vi "1A Interpret NMEA Sentence.vi"(11 "NMEA Sentence":string) -> ()   [LabVIEW 2013]
doc: "Interprets the NMEA 0813 sentences that we are using from our Airmar PB200 WeatherStation sensor.\nBy Jaime McCandless\nTODO: finish implementing NMEA sentences"
uses:
  <vilib>/regexp/Match Regular Expression.xnode
  2-Think/2 Globals/2 Global.vi
  2-Think/2 Typedefs/Velocity.ctl
  2-Think/2 Typedefs/apparent wind.ctl
  2-Think/2 Typedefs/pitch and roll.ctl
  2-Think/2 Typedefs/heading.ctl
  Data/TypeDefs/UTM Location.ctl
panel:
  in  "UTC Time Zone":i32=-5
  in  "Tab Control":T1(tab)
  out "GPS (GGA) Data":T2
  out "GPS (GLL) Data":T3
  out "GPGSA Data":T4
  out "UTC Time":timestamp
  out "Local Time":timestamp
  out "Lattitude (ddmm.mmmm)":dbl format="%_8g"
  out "Lattitude North/South":string
  out "Longitude (ddmm.mmmm)":dbl format="%_8g"
  out "Longitude East/West":string
  out "Speed over ground (knots)":dbl format="%_3g"
  out "Course over ground (degrees)":dbl format="%_4g"
  out "Magnetic Variation (degrees)":dbl format="%_4g"
  out "Variation East/West":string
  out "GPS (RMC) Data":T5 {"Course over ground (degrees)" format="%#.6g"; "Speed over ground (knots)" format="%#.6g"; "Magnetic Variation (degrees)" format="%#.6g"; "Longitude (ddmm.mmmm)" format="%#.6g"; "Lattitude (ddmm.mmmm)" format="%#.6g"}
  out "GPS Data Valid?":bool
  out "Robot UTM Location":T6 {"North" format="%#_10f"; "East" format="%#_8f"}
  out "GPS (VTG) Data":T7
  out "Heading":dbl
  out "Turn (ROT) Data":T8
  out "Meteorological Data":T9
  out "Theoretical true wind direction":T10(graph)
  out "Relative wind direction":cluster{dbl, "Filtered Value Out":dbl}(graph)
  out "Wind (MWV) Data, Theoretical":T11
  out "Wind (MWV) Data, Relative":T11
  out "Transducer (XDR) B Data":cluster{"Pitch (deg)":dbl, "Roll (deg)":dbl}
  out "Transducer (XDR) A Data":T12
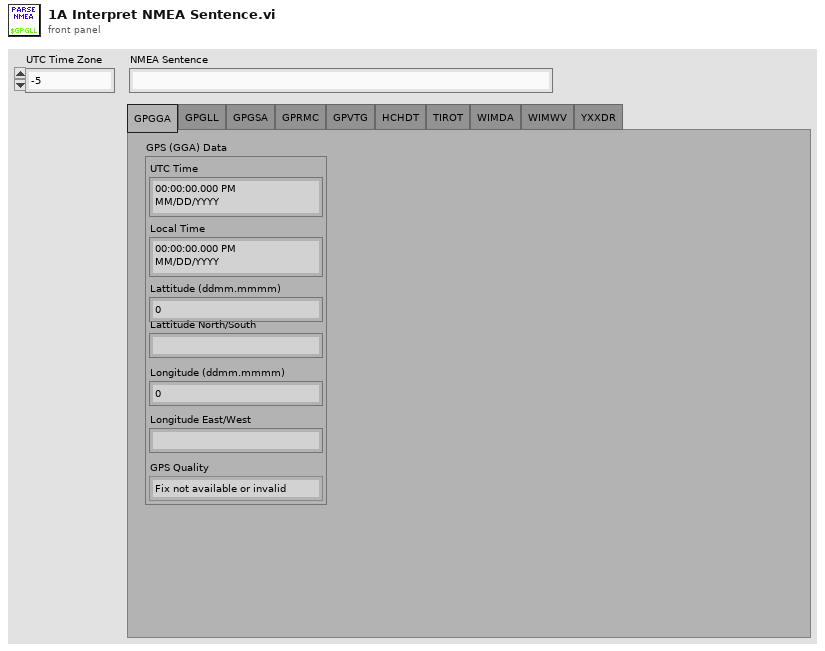
[diagram p1: front panel]
types:
  T1 = enum32{"GPGGA", "GPGLL", "GPGSA", "GPRMC", "GPVTG", "HCHDT", "TIROT", "WIMDA", "WIMWV", "YXXDR"}
  T2 = cluster{"UTC Time":timestamp, "Local Time":timestamp, "Lattitude (ddmm.mmmm)":dbl, "Lattitude North/South":string, "Longitude (ddmm.mmmm)":dbl, "Longitude East/West":string, "GPS Quality":enum16{"Fix not available or invalid", "GPS SPS Mode, fix valid", "Differential GPS, SPS Mode, fix valid", "GPS PPS Mode, fix valid", "Real Time Kinematic (RTK)", "Float RTK", "Estimated (dead reckoning) Mode", "Manual Input Mode", "Simulator Mode"}}
  T3 = cluster{"UTC Time":timestamp, "Local Time":timestamp, "Lattitude (ddmm.mmmm)":dbl, "Lattitude North/South":string, "Longitude (ddmm.mmmm)":dbl, "Longitude East/West":string, "GPS Mode":string, "GPS Data Valid?":bool}
  T4 = cluster{"Mode":string, "Fix Strength":i32, "Satellite IDs":i32[], "PDOP":dbl, "HDOP":dbl, "VDOP":dbl}
  T5 = cluster{"UTC Time":timestamp, "Local Time":timestamp, "Lattitude (ddmm.mmmm)":dbl, "Lattitude North/South":string, "Longitude (ddmm.mmmm)":dbl, "Longitude East/West":string, "Magnetic Variation (degrees)":dbl, "Variation East/West":string, "Speed over ground (knots)":dbl, "Course over ground (degrees)":dbl}
  T6 = typedef "UTM Location.ctl" = cluster{"UTM Zone":dbl, "Hemisphere":enum16{"North", "South"}, "East":dbl, "North":dbl}
  T7 = cluster{"Course Over Ground (True)":dbl, "Course Over Ground (Magnetic)":dbl, "Speed Over Ground (Knots)":dbl, "Speed Over Ground (km/hr)":dbl, "GPS Mode":string}
  T8 = cluster{"Rate of Turn (deg/min)":dbl, "Turn Rotation Data Valid?":bool}
  T9 = cluster{"Barometric Pressure (inches of mercury)":dbl, "Barometric Pressure (bars)":dbl, "Air temperature (degC)":dbl, "Relative humidity (%)":dbl, "Wind direction, True (deg)":dbl, "Wind direction, Magnetic (deg)":dbl, "Wind speed (knots)":dbl, "Wind speed (m/s)":dbl}
  T10 = cluster{"Robot\nHeading ":dbl, "Robot\nHeading ":dbl}
  T11 = cluster{"Angle relative to boat (deg)":dbl, "Wind Data Valid?":bool, "Wind speed (knots)":dbl, "True (T) or Relative (R)":string}
  T12 = cluster{"Calc. Relative Wind Chill (degC)":dbl, "Calc. Theoretical Wind Chill (degC)":dbl, "Calc. Heat Index (degC)":dbl, "Meas. Barometric Pressure (bars)":dbl}
  T13 = cluster{"second":i32, "minute":i32, "hour":i32, "day of month":i32, "month":i32, "year":i32, "day of week":i32, "day of year":i32, "is DST":i32}
  T14 = typedef "heading.ctl" = dbl
  T15 = typedef "Velocity.ctl" = cluster{"East":dbl, "North":dbl}
  T16 = typedef "apparent wind.ctl" = cluster{"Toward Fore":dbl, "Toward Starboard":dbl}
  T17 = typedef "pitch and roll.ctl" = cluster{"Pitch":dbl, "Roll":dbl}
  T18 = typedef "generalized sensor status.ctl" = cluster{"Sensor Connected":T19, "Sensor Initialized":T19, "Sensor OK":T19, "Latest Error String":string, "GPS Lock":T19}
  T19 = typedef "indicator LED.ctl" = bool
  T20 = cluster{"BoatVelocityInY":dbl, "BoatVelocityInX":dbl}
  T21 = cluster{"Robot\nHeading ":T14, "Robot\nHeading ":T14}
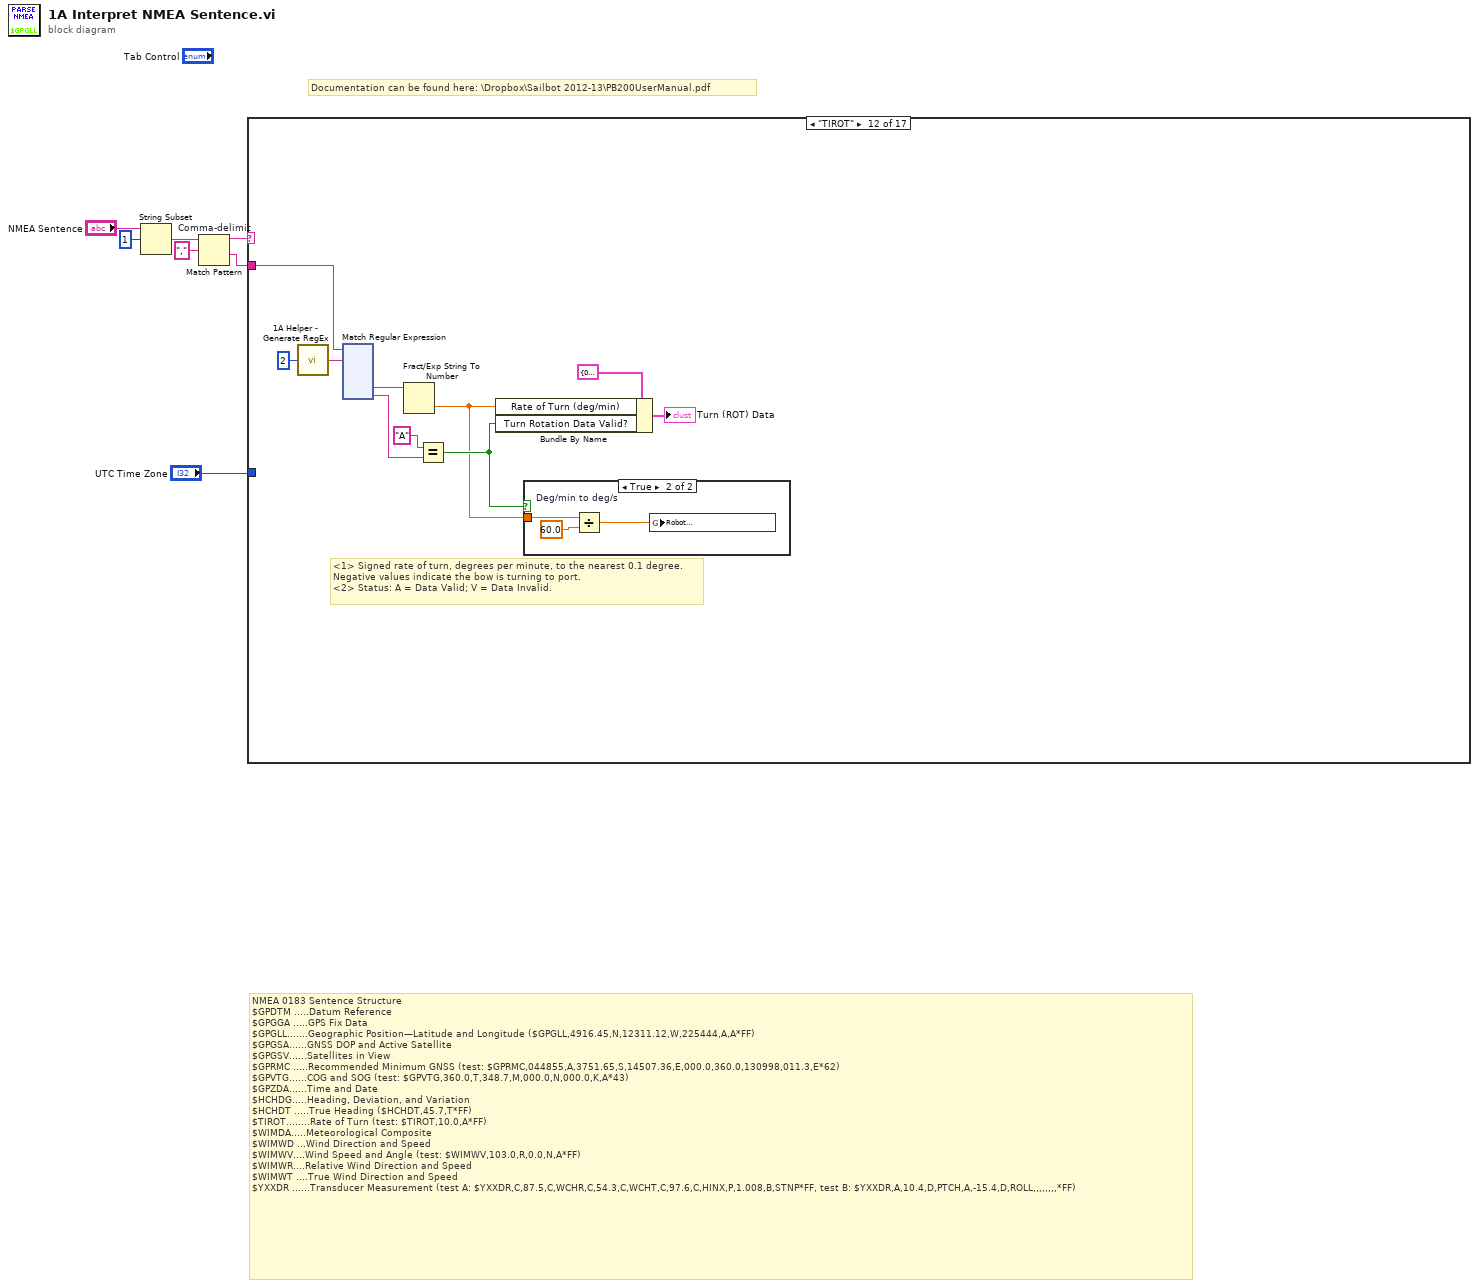
[diagram p0: block diagram]
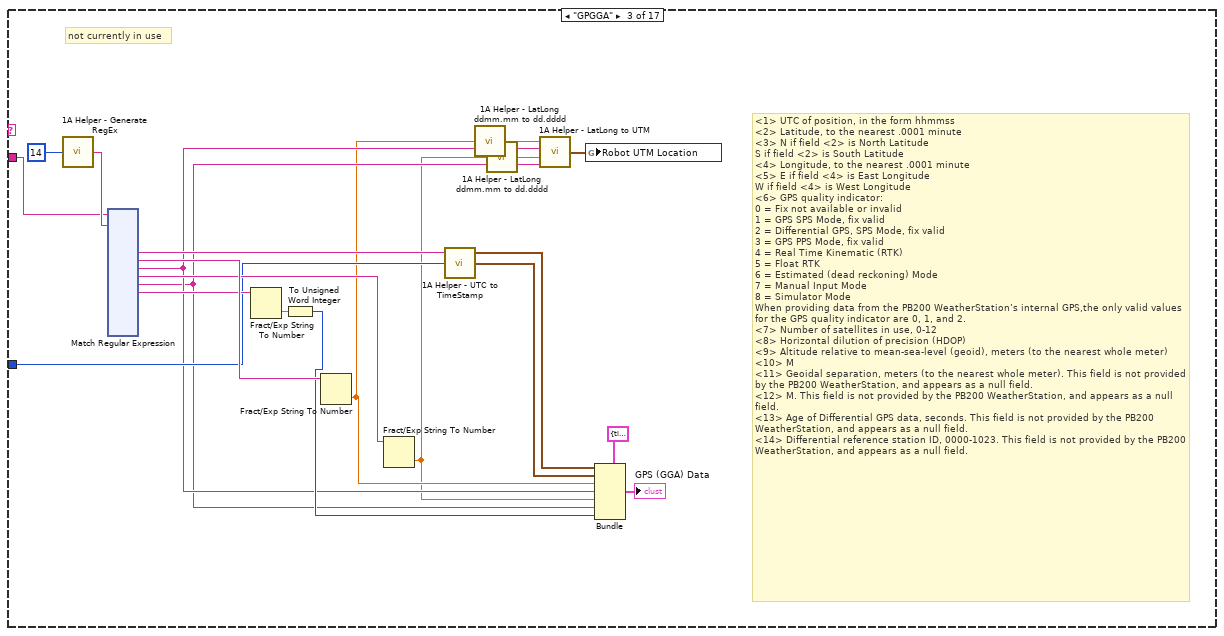
[diagram p4: hidden frame]
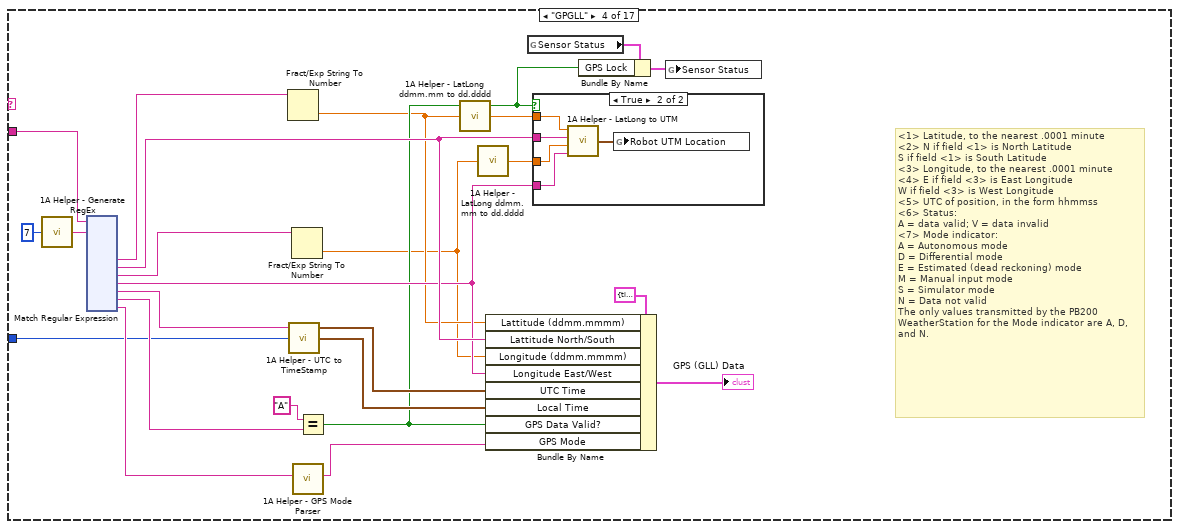
[diagram p5: hidden frame]
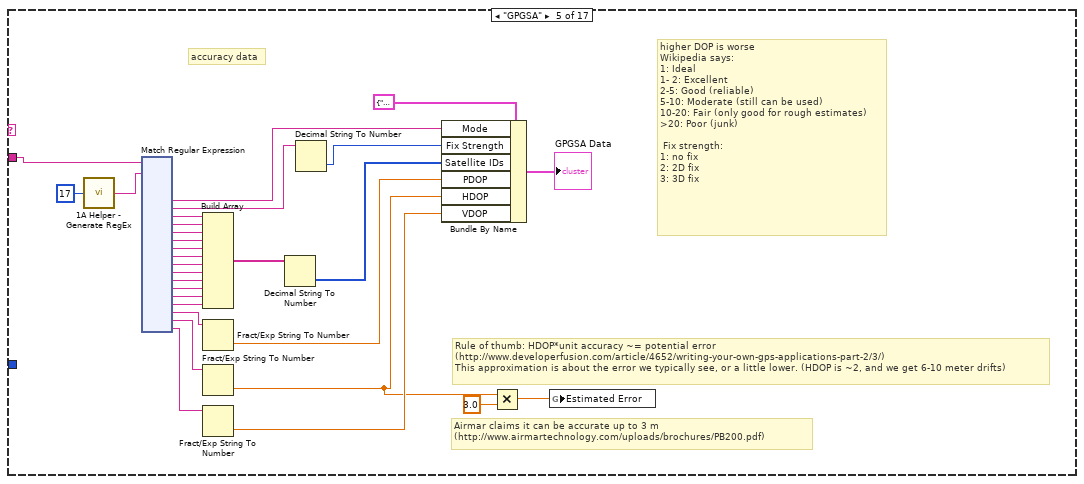
[diagram p7: hidden frame]
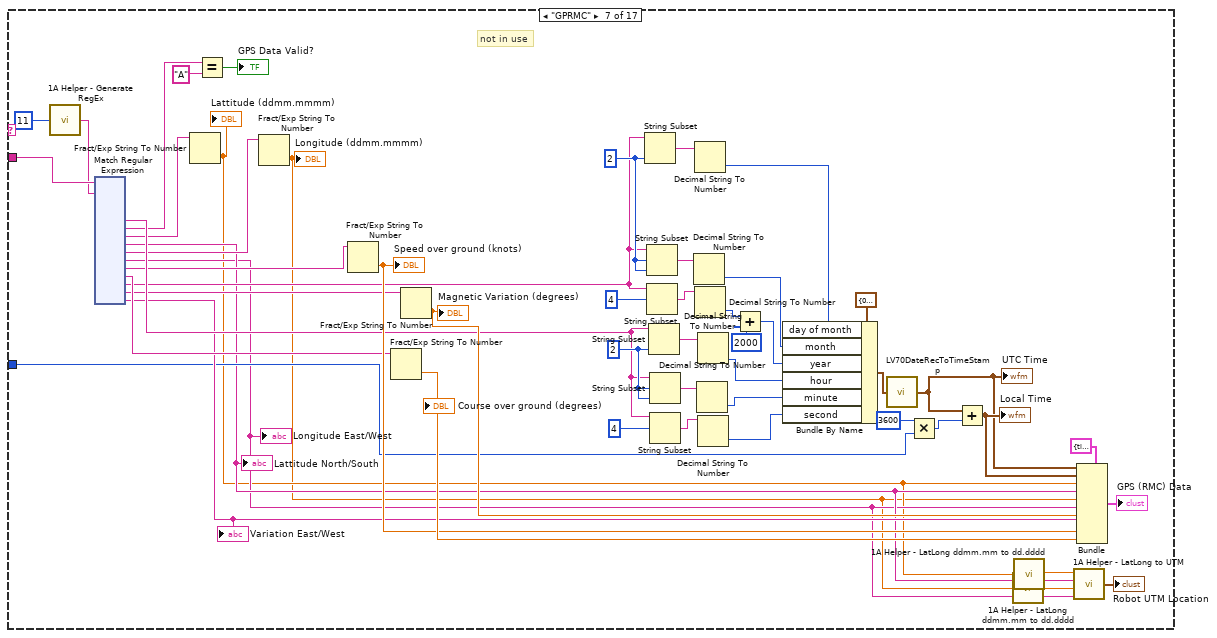
[diagram p9: hidden frame]
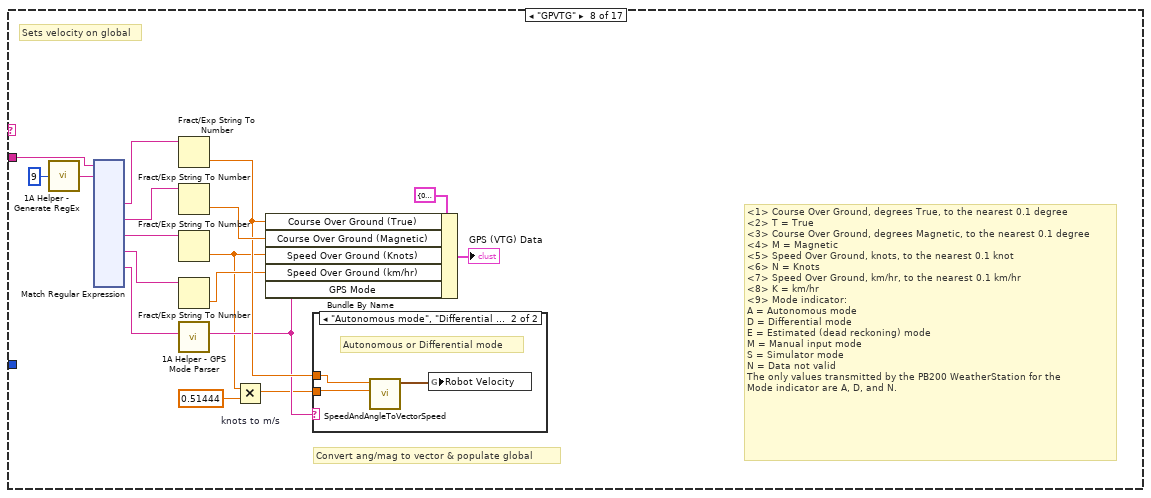
[diagram p10: hidden frame]
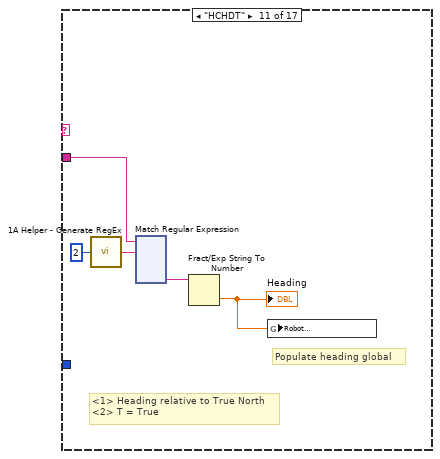
[diagram p14: hidden frame]
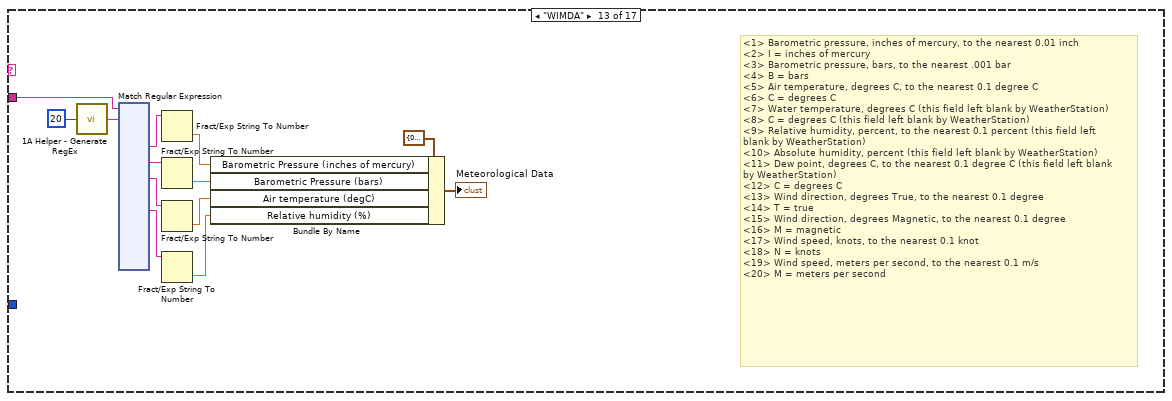
[diagram p16: hidden frame]
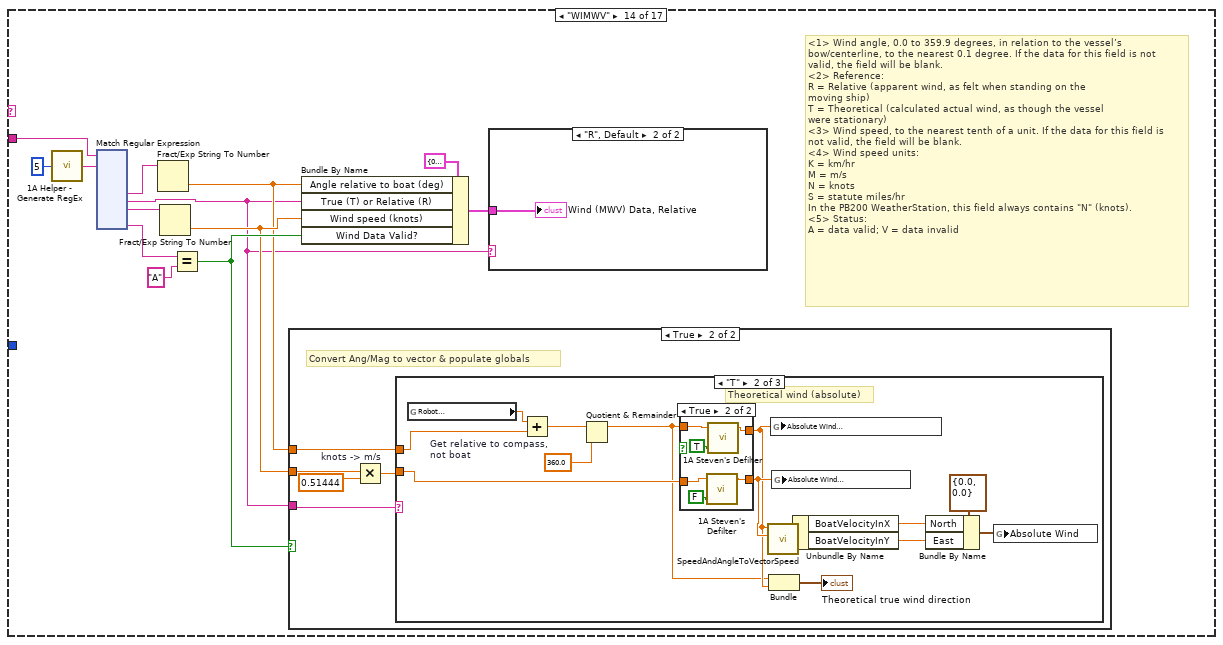
[diagram p17: hidden frame]
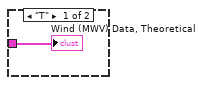
[diagram p18: hidden frame]
diagram:
  # "Documentation can be found here: \\Dropbox\\Sailbot 2012-13\\PB200UserManual.pdf"
  # "NMEA 0183 Sentence Structure\n$GPDTM .....Datum Reference\n$GPGGA .....GPS Fix Data\n$GPGLL.......Geographic Position—Latitude and Longitude ($GPGLL,4916.45,N,12311.12,W,225444,A,A*FF)\n$GPGSA......GNSS DOP and Active Satellite\n$GPGSV......Satellites in View\n$GPRMC .....Recommended Minimum GNSS (test: $GPRMC,044855,A,3751.65,S,14507.36,E,000.0,360.0,130998,011.3,E*62)\n$GPVTG......COG and SOG (test: $GPVTG,360.0,T,348.7,M,000.0,N,000.0,K,A*43)\n$GPZDA......Time and Date\n$HCHDG.....Heading, Deviation, and Variation\n$HCHDT .....True Heading ($HCHDT,45.7,T*FF)\n$TIROT........Rate of Turn (test: $TIROT,10.0,A*FF)\n$WIMDA.....Meteorological Composite\n$WIMWD ...Wind Direction and Speed\n$WIMWV....Wind Speed and Angle (test: $WIMWV,103.0,R,0.0,N,A*FF)\n$WIMWR....Relative Wind Direction and Speed\n$WIMWT ....True Wind Direction and Speed\n$YXXDR ......Transducer Measurement (test A: $YXXDR,C,87.5,C,WCHR,C,54.3,C,WCHT,C,97.6,C,HINX,P,1.008,B,STNP*FF, test B: $YXXDR,A,10.4,D,PTCH,A,-15.4,D,ROLL,,,,,,,,*FF)"
  n1 = String Subset(string="NMEA Sentence", offset (0)=1) -> (substring=w4:string)  [unwired: 1 in]
  n2 = Match Pattern "Comma-delimit"(string=w4, regular expression=",") -> (before substring=w5:string, after substring=w6:string)  [unwired: 1 in, 2 out]
  n3 = case shown="\"TIROT\"" w5 {
    tunnel: w6 -> [_ _ w26 w170 w329 _ w478 w647 _ _ w778 w900 w1031 w1170 _ _ w1329]
    tunnel: "UTC Time Zone" -> [_ _ w15 w162 _ _ w466 _ _ _ _ _ _ _ _ _ _]
    frame "", Default {
    }
    frame "GPDTM" {
      # "unimplemented"
    }
    frame "GPGGA" {
      # "not currently in use"
      # "<1> UTC of position, in the form hhmmss\n<2> Latitude, to the nearest .0001 minute\n<3> N if field <2> is North Latitude\nS if field <2> is South Latitude\n<4> Longitude, to the nearest .0001 minute\n<5> E if field <4> is East Longitude\nW if field <4> is West Longitude\n<6> GPS quality indicator:\n0 = Fix not available or invalid\n1 = GPS SPS Mode, fix valid\n2 = Differential GPS, SPS Mode, fix valid\n3 = GPS PPS Mode, fix valid\n4 = Real Time Kinematic (RTK)\n5 = Float RTK\n6 = Estimated (dead reckoning) Mode\n7 = Manual Input Mode\n8 = Simulator Mode\nWhen providing data from the PB200 WeatherStation’s internal GPS,the only valid values for the GPS quality indicator are 0, 1, and 2.\n<7> Number of satellites in use, 0-12\n<8> Horizontal dilution of precision (HDOP)\n<9> Altitude relative to mean-sea-level (geoid), meters (to the nearest whole meter)\n<10> M\n<11> Geoidal separation, meters (to the nearest whole meter). This field is not provided by the PB200 WeatherStation, and appears as a null field.\n<12> M. This field is not provided by the PB200 WeatherStation, and appears as a null field.\n<13> Age of Differential GPS data, seconds. This field is not provided by the PB200 WeatherStation, and appears as a null field.\n<14> Differential reference station ID, 0000-1023. This field is not provided by the PB200 WeatherStation, and appears as a null field."
      n4 = call "1A Helper - Generate RegEx.vi"("# Datums"=14) -> ("RegEx"=w27:string)
      n5 = xnode "Match Regular Expression"("input string"=w26, "regular expression"=w27) -> ("submatch 1"=w18:string, "submatch 2"=w24:string, "submatch 3"=w13:string, "submatch 4"=w23:string, "submatch 5"=w12:string, "submatch 6"=w22:string)  [unwired: 4 in, 10 out]
      n6 = Fract/Exp String To Number(string=w22) -> (number=w21:dbl)  [unwired: 3 in, 1 out]
      n7 = To Unsigned Word Integer(number=w21) -> (unsigned 16bit integer=w20:u16)
      n8 = Fract/Exp String To Number(string=w24) -> (number=w10:dbl)  [unwired: 3 in, 1 out]
      n9 = Fract/Exp String To Number(string=w23) -> (number=w8:dbl)  [unwired: 3 in, 1 out]
      n10 = call "1A Helper - UTC to TimeStamp.vi"("UTC Time Zone in"=w15, "UTC (hhmmss)"=w18) -> ("Local Time"=w16:timestamp, "UTC Time"=w17:timestamp)  [unwired: 2 in]
      n11 = call "1A Helper - LatLong ddmm.mm to dd.dddd.vi"("Lattitude/Longitude in ddmm.mmmm"=w10) -> ("Latitude/Longitude in dd.dddddd"=w11:dbl)
      n12 = call "1A Helper - LatLong ddmm.mm to dd.dddd.vi"("Lattitude/Longitude in ddmm.mmmm"=w8) -> ("Latitude/Longitude in dd.dddddd"=w9:dbl)
      n13 = call "1A Helper - LatLong to UTM.vi"("East/West"=w12, "Longitude"=w9, "North/South"=w13, "Latitude"=w11) -> ("Robot UTM Location"=w14:T6)
      n14 = global write "2 Global.vi" "Robot UTM Location"(w14) -> ()
      n15 = Bundle(cluster=T2 {"UTC Time"=timestamp(0 s since 1904-01-01), "Local Time"=timestamp(0 s since 1904-01-01), "Lattitude (ddmm.mmmm)"=0.0, "Lattitude North/South"="", "Longitude (ddmm.mmmm)"=0.0, "Longitude East/West"="", "GPS Quality"=enum."GPS SPS Mode, fix valid"} ("Cluster"), "UTC Time"=w17, "Local Time"=w16, "Lattitude (ddmm.mmmm)"=w10, "Lattitude North/South"=w13, "Longitude (ddmm.mmmm)"=w8, "Longitude East/West"=w12, "GPS Quality"=w20) -> (→"GPS (GGA) Data":T2)
    }
    frame "GPGLL" {
      # "<1> Latitude, to the nearest .0001 minute\n<2> N if field <1> is North Latitude\nS if field <1> is South Latitude\n<3> Longitude, to the nearest .0001 minute\n<4> E if field <3> is East Longitude\nW if field <3> is West Longitude\n<5> UTC of position, in the form hhmmss\n<6> Status:\nA = data valid; V = data invalid\n<7> Mode indicator:\nA = Autonomous mode\nD = Differential mode\nE = Estimated (dead reckoning) mode\nM = Manual input mode\nS = Simulator mode\nN = Data not valid\nThe only values transmitted by the PB200 WeatherStation for the Mode indicator are A, D, and N."
      n16 = call "1A Helper - Generate RegEx.vi"("# Datums"=7) -> ("RegEx"=w174:string)
      n17 = xnode "Match Regular Expression"("input string"=w170, "regular expression"=w174) -> ("submatch 1"=w173:string, "submatch 2"=w160:string, "submatch 3"=w172:string, "submatch 4"=w159:string, "submatch 5"=w169:string, "submatch 6"=w165:string, "submatch 7"=w171:string)  [unwired: 4 in, 5 out]
      n18 = Fract/Exp String To Number(string=w173) -> (number=w155:dbl)  [unwired: 3 in, 1 out]
      n19 = call "1A Helper - UTC to TimeStamp.vi"("UTC Time Zone in"=w162, "UTC (hhmmss)"=w169) -> ("Local Time"=w164:timestamp, "UTC Time"=w163:timestamp)  [unwired: 2 in]
      n20 = Fract/Exp String To Number(string=w172) -> (number=w153:dbl)  [unwired: 3 in, 1 out]
      n21 = call "1A Helper - GPS Mode Parser.vi"("GPS Mode (Char)"=w171) -> ("GPS Mode (Description)"=w167:string)  [unwired: 6 in]
      n22 = Equal?(x="A" ("y"), y=w165) -> (x = y?=w156:bool)
      n23 = call "1A Helper - LatLong ddmm.mm to dd.dddd.vi"("Lattitude/Longitude in ddmm.mmmm"=w155) -> ("Latitude/Longitude in dd.dddddd"=w154:dbl)
      n24 = call "1A Helper - LatLong ddmm.mm to dd.dddd.vi"("Lattitude/Longitude in ddmm.mmmm"=w153) -> ("Latitude/Longitude in dd.dddddd"=w152:dbl)
      n25 = Bundle By Name(cluster=T3 {"UTC Time"=timestamp(0 s since 1904-01-01), "Local Time"=timestamp(0 s since 1904-01-01), "Lattitude (ddmm.mmmm)"=0.0, "Lattitude North/South"="", "Longitude (ddmm.mmmm)"=0.0, "Longitude East/West"="", "GPS Mode"="", "GPS Data Valid?"=FALSE} ("Cluster"), "Lattitude (ddmm.mmmm)"=w155, "Lattitude North/South"=w160, "Longitude (ddmm.mmmm)"=w153, "Longitude East/West"=w159, "UTC Time"=w163, "Local Time"=w164, "GPS Data Valid?"=w156, "GPS Mode"=w167) -> (→"GPS (GLL) Data":T3)
      n26 = global read "2 Global.vi" "Sensor Status"() -> (w157:T18)
      n27 = case shown="True" w156 {
        tunnel: w154 -> [_ w180]
        tunnel: w160 -> [_ w179]
        tunnel: w152 -> [_ w178]
        tunnel: w159 -> [_ w177]
        frame False {
        }
        frame True {
          n28 = call "1A Helper - LatLong to UTM.vi"("East/West"=w177, "Longitude"=w178, "North/South"=w179, "Latitude"=w180) -> ("Robot UTM Location"=w176:T6)
          n29 = global write "2 Global.vi" "Robot UTM Location"(w176) -> ()
        }
      }
      n30 = Bundle By Name(cluster=w157, "GPS Lock"=w156) -> (w158:T18)
      n31 = global write "2 Global.vi" "Sensor Status"(w158) -> ()
    }
    frame "GPGSA" {
      # "Airmar claims it can be accurate up to 3 m\n(http://www.airmartechnology.com/uploads/brochures/PB200.pdf)"
      # "Rule of thumb: HDOP*unit accuracy ~= potential error\n(http://www.developerfusion.com/article/4652/writing-your-own-gps-applications-part-2/3/)\nThis approximation is about the error we typically see, or a little lower. (HDOP is ~2, and we get 6-10 meter drifts)"
      # "higher DOP is worse\nWikipedia says:\n1: Ideal\n1- 2: Excellent\n2-5: Good (reliable)\n5-10: Moderate (still can be used)\n10-20: Fair (only good for rough estimates)\n>20: Poor (junk)\n\n Fix strength: \n1: no fix\n2: 2D fix\n3: 3D fix"
      # "accuracy data"
      n32 = call "1A Helper - Generate RegEx.vi"("# Datums"=17) -> ("RegEx"=w328:string)
      n33 = xnode "Match Regular Expression"("input string"=w329, "regular expression"=w328) -> ("submatch 1"=w325:string, "submatch 2"=w324:string, "submatch 3"=w322:string, "submatch 4"=w321:string, "submatch 5"=w320:string, "submatch 6"=w319:string, "submatch 7"=w318:string, "submatch 8"=w317:string, "submatch 9"=w316:string, "submatch 10"=w315:string, "submatch 11"=w314:string, "submatch 12"=w313:string, "submatch 13"=w312:string, "submatch 14"=w311:string, "submatch 15"=w308:string, "submatch 16"=w306:string, "submatch 17"=w305:string)  [unwired: 4 in, 5 out]
      n34 = Build Array(w322, w321, w320, w319, w318, w317, w316, w315, w314, w313, w312, w311) -> (w310:string[])
      n35 = Fract/Exp String To Number(string=w308) -> (number=w307:dbl)  [unwired: 3 in, 1 out]
      n36 = Fract/Exp String To Number(string=w306) -> (number=w302:dbl)  [unwired: 3 in, 1 out]
      n37 = Fract/Exp String To Number(string=w305) -> (number=w304:dbl)  [unwired: 3 in, 1 out]
      n38 = Decimal String To Number(string=w310) -> (number=w309:i32[])  [unwired: 2 in, 1 out]
      n39 = Decimal String To Number(string=w324) -> (number=w323:i32)  [unwired: 2 in, 1 out]
      n40 = Bundle By Name(cluster=T4 {"Mode"="", "Fix Strength"=0, "Satellite IDs"=[], "PDOP"=0.0, "HDOP"=0.0, "VDOP"=0.0} ("GPGSA Data"), "Mode"=w325, "Fix Strength"=w323, "Satellite IDs"=w309, "PDOP"=w307, "HDOP"=w302, "VDOP"=w304) -> (→"GPGSA Data":T4)
      n41 = Multiply(x=w302, y=3.0) -> (x*y=w300:dbl)
      n42 = global write "2 Global.vi" "Estimated Error"(w300) -> ()
    }
    frame "GPGSV" {
      # "unimplemented"
    }
    frame "GPRMC" {
      w496 = 2 ("length (rest)")
      w486 = 2 ("length (rest)")
      # "not in use"
      n43 = call "1A Helper - Generate RegEx.vi"("# Datums"=11) -> ("RegEx"=w468:string)
      n44 = xnode "Match Regular Expression"("input string"=w478, "regular expression"=w468) -> ("submatch 1"=w477:string, "submatch 2"=w476:string, "submatch 3"=w475:string, "submatch 4"=w465:string, "submatch 5"=w474:string, "submatch 6"=w464:string, "submatch 7"=w473:string, "submatch 8"=w472:string, "submatch 9"=w471:string, "submatch 10"=w470:string, "submatch 11"=w469:string)  [unwired: 4 in, 5 out]
      "Lattitude North/South" <- w465
      "Longitude East/West" <- w464
      "Variation East/West" <- w469
      n45 = Fract/Exp String To Number(string=w475) -> (number=w461:dbl)  [unwired: 3 in, 1 out]
      "Lattitude (ddmm.mmmm)" <- w461
      n46 = Equal?(x=w476, y="A") -> (x = y?=→"GPS Data Valid?":bool)
      n47 = Fract/Exp String To Number(string=w474) -> (number=w459:dbl)  [unwired: 3 in, 1 out]
      "Longitude (ddmm.mmmm)" <- w459
      n48 = Fract/Exp String To Number(string=w473) -> (number=w506:dbl)  [unwired: 3 in, 1 out]
      "Speed over ground (knots)" <- w506
      n49 = Fract/Exp String To Number(string=w472) -> (number=w507:dbl)  [unwired: 3 in, 1 out]
      "Course over ground (degrees)" <- w507
      n50 = Fract/Exp String To Number(string=w470) -> (number=w505:dbl)  [unwired: 3 in, 1 out]
      "Magnetic Variation (degrees)" <- w505
      n51 = String Subset(string=w471, length (rest)=w496) -> (substring=w497:string)  [unwired: 1 in]
      n52 = String Subset(string=w471, offset (0)=w496, length (rest)=w496) -> (substring=w495:string)
      n53 = String Subset(string=w471, offset (0)=4) -> (substring=w493:string)  [unwired: 1 in]
      n54 = String Subset(string=w477, length (rest)=w486) -> (substring=w482:string)  [unwired: 1 in]
      n55 = String Subset(string=w477, offset (0)=w486, length (rest)=w486) -> (substring=w488:string)
      n56 = String Subset(string=w477, offset (0)=4) -> (substring=w490:string)  [unwired: 1 in]
      n57 = Decimal String To Number(string=w495) -> (number=w499:i32)  [unwired: 2 in, 1 out]
      n58 = Decimal String To Number(string=w497) -> (number=w498:i32)  [unwired: 2 in, 1 out]
      n59 = Decimal String To Number(string=w493) -> (number=w500:i32)  [unwired: 2 in, 1 out]
      n60 = Decimal String To Number(string=w488) -> (number=w487:i32)  [unwired: 2 in, 1 out]
      n61 = Decimal String To Number(string=w482) -> (number=w485:i32)  [unwired: 2 in, 1 out]
      n62 = Decimal String To Number(string=w490) -> (number=w491:i32)  [unwired: 2 in, 1 out]
      n63 = Add(x=w500, y=2000) -> (x+y=w502:i32)
      n64 = Bundle By Name(cluster=T13 {"second"=0, "minute"=0, "hour"=0, "day of month"=0, "month"=0, "year"=0, "day of week"=0, "day of year"=0, "is DST"=0} ("date time rec"), "day of month"=w498, "month"=w499, "year"=w502, "hour"=w485, "minute"=w487, "second"=w491) -> (w483:T13)
      n65 = call <vilib>:"LV70DateRecToTimeStamp.vi"("date time rec"=w483) -> ("Time Stamp"=w503:timestamp)
      "UTC Time" <- w503
      n66 = Multiply(x=3600 ("number"), y=w466) -> (x*y=w467:i32)
      n67 = Add(x=w503, y=w467) -> (x+y=w504:timestamp)
      "Local Time" <- w504
      n68 = call "1A Helper - LatLong ddmm.mm to dd.dddd.vi"("Lattitude/Longitude in ddmm.mmmm"=w459) -> ("Latitude/Longitude in dd.dddddd"=w460:dbl)
      n69 = call "1A Helper - LatLong ddmm.mm to dd.dddd.vi"("Lattitude/Longitude in ddmm.mmmm"=w461) -> ("Latitude/Longitude in dd.dddddd"=w462:dbl)
      n70 = call "1A Helper - LatLong to UTM.vi"("East/West"=w464, "Longitude"=w460, "North/South"=w465, "Latitude"=w462) -> ("Robot UTM Location"=→"Robot UTM Location":T6)
      n71 = Bundle(cluster=T5 {"UTC Time"=timestamp(0 s since 1904-01-01), "Local Time"=timestamp(0 s since 1904-01-01), "Lattitude (ddmm.mmmm)"=0.0, "Lattitude North/South"="", "Longitude (ddmm.mmmm)"=0.0, "Longitude East/West"="", "Magnetic Variation (degrees)"=0.0, "Variation East/West"="", "Speed over ground (knots)"=0.0, "Course over ground (degrees)"=0.0} ("Cluster"), "UTC Time"=w503, "Local Time"=w504, "Lattitude (ddmm.mmmm)"=w461, "Lattitude North/South"=w465, "Longitude (ddmm.mmmm)"=w459, "Longitude East/West"=w464, "Magnetic Variation (degrees)"=w505, "Variation East/West"=w469, "Speed over ground (knots)"=w506, "Course over ground (degrees)"=w507) -> (→"GPS (RMC) Data":T5)
    }
    frame "GPVTG" {
      # "Convert ang/mag to vector & populate global"
      # "Sets velocity on global"
      # "<1> Course Over Ground, degrees True, to the nearest 0.1 degree\n<2> T = True\n<3> Course Over Ground, degrees Magnetic, to the nearest 0.1 degree\n<4> M = Magnetic\n<5> Speed Over Ground, knots, to the nearest 0.1 knot\n<6> N = Knots\n<7> Speed Over Ground, km/hr, to the nearest 0.1 km/hr\n<8> K = km/hr\n<9> Mode indicator:\nA = Autonomous mode\nD = Differential mode\nE = Estimated (dead reckoning) mode\nM = Manual input mode\nS = Simulator mode\nN = Data not valid\nThe only values transmitted by the PB200 WeatherStation for the\nMode indicator are A, D, and N."
      n72 = call "1A Helper - Generate RegEx.vi"("# Datums"=9) -> ("RegEx"=w648:string)
      n73 = xnode "Match Regular Expression"("input string"=w647, "regular expression"=w648) -> ("submatch 1"=w644:string, "submatch 3"=w643:string, "submatch 5"=w641:string, "submatch 7"=w640:string, "submatch 9"=w639:string)  [unwired: 4 in, 11 out]
      n74 = Fract/Exp String To Number(string=w644) -> (number=w638:dbl)  [unwired: 3 in, 1 out]
      n75 = Fract/Exp String To Number(string=w643) -> (number=w642:dbl)  [unwired: 3 in, 1 out]
      n76 = Fract/Exp String To Number(string=w641) -> (number=w635:dbl)  [unwired: 3 in, 1 out]
      n77 = Fract/Exp String To Number(string=w640) -> (number=w637:dbl)  [unwired: 3 in, 1 out]
      n78 = call "1A Helper - GPS Mode Parser.vi"("GPS Mode (Char)"=w639) -> ("GPS Mode (Description)"=w636:string)  [unwired: 6 in]
      n79 = Multiply "knots to m/s"(x=w635, y=0.51444) -> (x*y=w634:dbl)
      n80 = Bundle By Name(cluster=T7 {"Course Over Ground (True)"=0.0, "Course Over Ground (Magnetic)"=0.0, "Speed Over Ground (Knots)"=0.0, "Speed Over Ground (km/hr)"=0.0, "GPS Mode"=""} ("GPS (VTG) Data 2"), "Course Over Ground (True)"=w638, "Course Over Ground (Magnetic)"=w642, "Speed Over Ground (Knots)"=w635, "Speed Over Ground (km/hr)"=w637, "GPS Mode"=w636) -> (→"GPS (VTG) Data":T7)
      n81 = case shown="\"Autonomous mode\", \"Differential mode\"" w636 {
        tunnel: w638 -> [_ w652]
        tunnel: w634 -> [_ w651]
        frame "Data not valid", Default {
          # "Data not valid"
        }
        frame "Autonomous mode", "Differential mode" {
          # "Autonomous or Differential mode"
          n82 = call "SpeedAndAngleToVectorSpeed.vi"("BoatSpeed (m/s)"=w651, "RobotHeading (deg)"=w652) -> ("BoatVectorVelocity"=w650:T20)  [unwired: 9 in]
          n83 = global write "2 Global.vi" "Robot Velocity"(w650) -> ()
        }
      }
    }
    frame "GPZDA" {
      # "<1> UTC time of day, in the form hhmmss\n<2> UTC day, 01 to 31\n<3> UTC month, 01 to 12\n<4> UTC year (four digits, e.g. 2006)\n<5> Local time zone hours, 00 to +/-13 hrs\n<6> Local time zone minutes, 00 to +59"
    }
    frame "HCHDG " {
      # "<1> Magnetic sensor heading, degrees, to the nearest 0.1 degree.\n<2> Magnetic deviation, degrees east or west, to the nearest 0.1 degree.\n<3> E if field <2> is degrees East\nW if field <2> is degrees West\n<4> Magnetic variation, degrees east or west, to the nearest 0.1 degree.\n<5> E if field <4> is degrees East\nW if field <4> is degrees West"
    }
    frame "HCHDT" {
      # "Populate heading global"
      # "<1> Heading relative to True North\n<2> T = True"
      n84 = call "1A Helper - Generate RegEx.vi"("# Datums"=2) -> ("RegEx"=w779:string)
      n85 = xnode "Match Regular Expression"("input string"=w778, "regular expression"=w779) -> ("submatch 1"=w777:string)  [unwired: 4 in, 5 out]
      n86 = Fract/Exp String To Number(string=w777) -> (number=w776:dbl)  [unwired: 3 in, 1 out]
      "Heading" <- w776
      n87 = global write "2 Global.vi" "Robot\nHeading"(w776) -> ()
    }
    frame "TIROT" {
      # "<1> Signed rate of turn, degrees per minute, to the nearest 0.1 degree.\nNegative values indicate the bow is turning to port.\n<2> Status: A = Data Valid; V = Data Invalid."
      n88 = call "1A Helper - Generate RegEx.vi"("# Datums"=2) -> ("RegEx"=w902:string)
      n89 = xnode "Match Regular Expression"("input string"=w900, "regular expression"=w902) -> ("submatch 1"=w901:string, "submatch 2"=w896:string)  [unwired: 4 in, 5 out]
      n90 = Fract/Exp String To Number(string=w901) -> (number=w894:dbl)  [unwired: 3 in, 1 out]
      n91 = Equal?(x="A" ("y"), y=w896) -> (x = y?=w895:bool)
      n92 = Bundle By Name(cluster=T8 {"Rate of Turn (deg/min)"=0.0, "Turn Rotation Data Valid?"=TRUE} ("Turn (ROT) Data 2"), "Rate of Turn (deg/min)"=w894, "Turn Rotation Data Valid?"=w895) -> (→"Turn (ROT) Data":T8)
      n93 = case shown="True" w895 {
        tunnel: w894 -> [_ w905]
        frame False {
        }
        frame True {
          n94 = Divide "Deg/min to deg/s"(x=w905, y=60.0) -> (x/y=w906:dbl)
          n95 = global write "2 Global.vi" "Robot\nRate of Turn"(w906) -> ()
        }
      }
    }
    frame "WIMDA" {
      # "<1> Barometric pressure, inches of mercury, to the nearest 0.01 inch\n<2> I = inches of mercury\n<3> Barometric pressure, bars, to the nearest .001 bar\n<4> B = bars\n<5> Air temperature, degrees C, to the nearest 0.1 degree C\n<6> C = degrees C\n<7> Water temperature, degrees C (this field left blank by WeatherStation)\n<8> C = degrees C (this field left blank by WeatherStation)\n<9> Relative humidity, percent, to the nearest 0.1 percent (this field left\nblank by WeatherStation)\n<10> Absolute humidity, percent (this field left blank by WeatherStation)\n<11> Dew point, degrees C, to the nearest 0.1 degree C (this field left blank\nby WeatherStation)\n<12> C = degrees C\n<13> Wind direction, degrees True, to the nearest 0.1 degree\n<14> T = true\n<15> Wind direction, degrees Magnetic, to the nearest 0.1 degree\n<16> M = magnetic\n<17> Wind speed, knots, to the nearest 0.1 knot\n<18> N = knots\n<19> Wind speed, meters per second, to the nearest 0.1 m/s\n<20> M = meters per second"
      n96 = call "1A Helper - Generate RegEx.vi"("# Datums"=20) -> ("RegEx"=w1032:string)
      n97 = xnode "Match Regular Expression"("input string"=w1031, "regular expression"=w1032) -> ("submatch 1"=w1025:string, "submatch 3"=w1024:string, "submatch 5"=w1023:string, "submatch 9"=w1022:string)  [unwired: 4 in, 17 out]
      n98 = Fract/Exp String To Number(string=w1025) -> (number=w1029:dbl)  [unwired: 3 in, 1 out]
      n99 = Fract/Exp String To Number(string=w1024) -> (number=w1028:dbl)  [unwired: 3 in, 1 out]
      n100 = Fract/Exp String To Number(string=w1023) -> (number=w1027:dbl)  [unwired: 3 in, 1 out]
      n101 = Fract/Exp String To Number(string=w1022) -> (number=w1026:dbl)  [unwired: 3 in, 1 out]
      n102 = Bundle By Name(cluster=T9 {"Barometric Pressure (inches of mercury)"=0.0, "Barometric Pressure (bars)"=0.0, "Air temperature (degC)"=0.0, "Relative humidity (%)"=0.0, "Wind direction, True (deg)"=0.0, "Wind direction, Magnetic (deg)"=0.0, "Wind speed (knots)"=0.0, "Wind speed (m/s)"=0.0} ("Meteorological Data"), "Barometric Pressure (inches of mercury)"=w1029, "Barometric Pressure (bars)"=w1028, "Air temperature (degC)"=w1027, "Relative humidity (%)"=w1026) -> (→"Meteorological Data":T9)
    }
    frame "WIMWV" {
      # "<1> Wind angle, 0.0 to 359.9 degrees, in relation to the vessel’s\nbow/centerline, to the nearest 0.1 degree. If the data for this field is not\nvalid, the field will be blank.\n<2> Reference:\nR = Relative (apparent wind, as felt when standing on the\nmoving ship)\nT = Theoretical (calculated actual wind, as though the vessel\nwere stationary)\n<3> Wind speed, to the nearest tenth of a unit. If the data for this field is\nnot valid, the field will be blank.\n<4> Wind speed units:\nK = km/hr\nM = m/s\nN = knots\nS = statute miles/hr\nIn the PB200 WeatherStation, this field always contains \"N\" (knots).\n<5> Status:\nA = data valid; V = data invalid"
      n103 = call "1A Helper - Generate RegEx.vi"("# Datums"=5) -> ("RegEx"=w1173:string)
      n104 = xnode "Match Regular Expression"("input string"=w1170, "regular expression"=w1173) -> ("submatch 1"=w1172:string, "submatch 2"=w1162:string, "submatch 3"=w1167:string, "submatch 5"=w1166:string)  [unwired: 4 in, 6 out]
      n105 = Fract/Exp String To Number(string=w1172) -> (number=w1163:dbl)  [unwired: 3 in, 1 out]
      n106 = Fract/Exp String To Number(string=w1167) -> (number=w1164:dbl)  [unwired: 3 in, 1 out]
      n107 = Equal?(x=w1166, y="A") -> (x = y?=w1165:bool)
      n108 = case shown="True" w1165 {
        tunnel: w1164 -> [_ w1178]
        tunnel: w1163 -> [_ w1181]
        tunnel: w1162 -> [_ w1180]
        frame False {
        }
        frame True {
          # "Convert Ang/Mag to vector & populate globals"
          n109 = Multiply "knots -> m/s"(x=w1178, y=0.51444) -> (x*y=w1179:dbl)
          n110 = case shown="\"T\"" w1180 {
            tunnel: w1179 -> [_ w1186 w1204]
            tunnel: w1181 -> [_ w1189 w1205]
            frame "", Default {
            }
            frame "T" {
              # "Theoretical wind (absolute)"
              n111 = global read "2 Global.vi" "Robot\nHeading"() -> (w1190:T14)
              n112 = Add "Get relative to compass, not boat"(x=w1190, y=w1189) -> (x+y=w1188:T14)
              n113 = Quotient & Remainder(x=w1188, y=T14 360.0) -> (x-y*floor(x/y)=w1183:T14)  [unwired: 1 out]
              n114 = case shown="True" {
                selector: _ -> [_ _]
                tunnel: [w1196 w1203] -> w1185
                tunnel: w1186 -> [w1196 w1202]
                tunnel: w1183 -> [w1197 w1201]
                tunnel: [w1197 w1200] -> w1184
                frame False {
                }
                frame True {
                  n115 = call "1A Steven's Defilter.vi"("Angle?(F)"=FALSE, "Value In"=w1202) -> ("Filtered Value Out"=w1203:dbl)  [unwired: 3 in]
                  n116 = call "1A Steven's Defilter.vi"("Angle?(F)"=TRUE, "Value In"=w1201) -> ("Filtered Value Out"=w1200:dbl)  [unwired: 3 in]
                }
              }
              n117 = call "SpeedAndAngleToVectorSpeed.vi"("BoatSpeed (m/s)"=w1185, "RobotHeading (deg)"=w1184) -> ("BoatVectorVelocity"=w1195:T20)  [unwired: 9 in]
              n118 = Bundle("Robot\nHeading"=w1183, "Robot\nHeading"=w1184) -> (→"Theoretical true wind direction":T21)  [unwired: 1 in]
              n119 = global write "2 Global.vi" "Absolute Wind\nDirection (º)"(w1184) -> ()
              n120 = global write "2 Global.vi" "Absolute Wind\nSpeed"(w1185) -> ()
              n121 = Unbundle By Name(w1195) -> ("BoatVelocityInX"=w1193:dbl, "BoatVelocityInY"=w1192:dbl)
              n122 = Bundle By Name(cluster=T15 {"East"=0.0, "North"=0.0} ("Absolute Wind"), "North"=w1193, "East"=w1192) -> (w1194:T15)
              n123 = global write "2 Global.vi" "Absolute Wind"(w1194) -> ()
            }
            frame "R" {
              # "Relative wind (apparent)"
              n124 = Bundle(w1205, w1205) -> (→"Relative wind direction":cluster{dbl, dbl})  [unwired: 1 in]
              n125 = global write "2 Global.vi" "Apparent Wind\nDirection (º)"(w1205) -> ()
              n126 = call "SpeedAndAngleToVectorSpeed.vi"("BoatSpeed (m/s)"=w1204, "RobotHeading (deg)"=w1205) -> ("BoatVectorVelocity"=w1207:T20)  [unwired: 9 in]
              n127 = global write "2 Global.vi" "Apparent Wind\nSpeed"(w1204) -> ()
              n128 = Unbundle By Name(w1207) -> ("BoatVelocityInX"=w1210:dbl, "BoatVelocityInY"=w1211:dbl)
              n129 = Bundle By Name(cluster=T16 {"Toward Fore"=0.0, "Toward Starboard"=0.0} ("Apparent Wind"), "Toward Fore"=w1210, "Toward Starboard"=w1211) -> (w1209:T16)
              n130 = global write "2 Global.vi" "Apparent Wind"(w1209) -> ()
            }
          }
        }
      }
      n131 = Bundle By Name(cluster=T11 {"Angle relative to boat (deg)"=0.0, "Wind Data Valid?"=TRUE, "Wind speed (knots)"=0.0, "True (T) or Relative (R)"=""} ("Wind (MWV) Data 2"), "Angle relative to boat (deg)"=w1163, "True (T) or Relative (R)"=w1162, "Wind speed (knots)"=w1164, "Wind Data Valid?"=w1165) -> (w1169:T11)
      n132 = case shown="\"R\", Default" w1162 {
        tunnel: w1169 -> [w1175 w1176]
        frame "T" {
          "Wind (MWV) Data, Theoretical" <- w1175
        }
        frame "R", Default {
          "Wind (MWV) Data, Relative" <- w1176
        }
      }
    }
    frame "WIMWR" {
    }
    frame "WIMWT" {
    }
    frame "YXXDR" {
      n133 = String Subset(string=w1329, length (rest)=1 ("length (rest)")) -> (substring=w1330:string)  [unwired: 1 in]
      n134 = case shown="\"A\"" w1330 {
        tunnel: w1329 -> [_ w1332 w1471]
        frame "", Default {
        }
        frame "A" {
          # "TYPE B:\n<1> A = angular displacement\n<2> Pitch: oscillation of vessel about its latitudinal axis. Bow moving up is positive. Value reported to the nearest 0.1 degree.\n<3> D = degrees\n<4> PTCH (ID indicating pitch of vessel)\n<5> A = angular displacement\n<6> Roll: oscillation of vessel about its longitudinal axis. Roll to the starboard is positive. Value reported to the nearest 0.1 degree.\n<7> D = degrees\n<8> ROLL (ID indicating roll of vessel)\n<9> Not used\n<10> Not used\n<11> Not used\n<12> Not used\n<13> Not used\n<14> Not used\n<15> Not used\n<16> Not used"
          n135 = call "1A Helper - Generate RegEx.vi"("# Datums"=8) -> ("RegEx"=w1336:string)
          n136 = xnode "Match Regular Expression"("input string"=w1332, "regular expression"=w1336) -> ("submatch 2"=w1334:string, "submatch 6"=w1333:string)  [unwired: 4 in, 19 out]
          n137 = Fract/Exp String To Number(string=w1334) -> (number=w1338:dbl)  [unwired: 3 in, 1 out]
          n138 = Fract/Exp String To Number(string=w1333) -> (number=w1337:dbl)  [unwired: 3 in, 1 out]
          n139 = Bundle By Name(cluster=cluster{"Pitch (deg)":dbl, "Roll (deg)":dbl} {"Pitch (deg)"=103.0, "Roll (deg)"=103.0} ("Transducer (XDR) B Data 2"), "Pitch (deg)"=w1338, "Roll (deg)"=w1337) -> (→"Transducer (XDR) B Data":cluster{"Pitch (deg)":dbl, "Roll (deg)":dbl})
          n140 = Bundle By Name(cluster=T17 {"Pitch"=0.0, "Roll"=0.0} ("Robot Pitch/Roll"), "Pitch"=w1338, "Roll"=w1337) -> (w1339:T17)
          n141 = global write "2 Global.vi" "Robot Pitch/Roll"(w1339) -> ()
        }
        frame "C" {
          # "TYPE A:\n<1> C = temperature\n<2> Calculated “relative” wind chill temperature, degrees Celsius, to the nearest 0.1 degree\n<3> C = degrees C\n<4> WCHR (ID indicating relative wind chill)\n<5> C = temperature\n<6> Calculated “theoretical” wind chill temperature, degrees Celsius, to the nearest 0.1 degree\n<7> C = degrees C\n<8> WCHT (ID indicating theoretical wind chill)\n<9> C = temperature\n<10> Calculated heat index, degrees Celsius, to the nearest 0.1 degree (this field left blank by WeatherStation)\n<11> C = degrees C\n<12> HINX (ID indicating heat index)\n<13> P = pressure\n<14> Actual measured barometric pressure, or \"station pressure\", bars, to the nearest 0.001 bar\n<15> B = bars\n<16> STNP (ID indicating station pressure)"
          n142 = call "1A Helper - Generate RegEx.vi"("# Datums"=16) -> ("RegEx"=w1477:string)
          n143 = xnode "Match Regular Expression"("input string"=w1471, "regular expression"=w1477) -> ("submatch 2"=w1475:string, "submatch 6"=w1474:string, "submatch 10"=w1473:string, "submatch 14"=w1472:string)  [unwired: 4 in, 17 out]
          n144 = Fract/Exp String To Number(string=w1475) -> (number=w1481:dbl)  [unwired: 3 in, 1 out]
          n145 = Fract/Exp String To Number(string=w1474) -> (number=w1480:dbl)  [unwired: 3 in, 1 out]
          n146 = Fract/Exp String To Number(string=w1473) -> (number=w1479:dbl)  [unwired: 3 in, 1 out]
          n147 = Fract/Exp String To Number(string=w1472) -> (number=w1478:dbl)  [unwired: 3 in, 1 out]
          n148 = Bundle By Name(cluster=T12 {"Calc. Relative Wind Chill (degC)"=0.0, "Calc. Theoretical Wind Chill (degC)"=0.0, "Calc. Heat Index (degC)"=0.0, "Meas. Barometric Pressure (bars)"=0.0} ("Transducer (XDR) A Data 2"), "Calc. Relative Wind Chill (degC)"=w1481, "Calc. Theoretical Wind Chill (degC)"=w1480, "Calc. Heat Index (degC)"=w1479, "Meas. Barometric Pressure (bars)"=w1478) -> (→"Transducer (XDR) A Data":T12)
        }
      }
    }
  }
